vi "exec.vi"(8 "error in (no error)":errorcluster, 9 "Save Data":bool, 10 "VISA":refnum<visa-resource-name>, 11 "ElectrometerController in":refnum<class "ElectrometerController.lvclass">) -> (0 "error out":errorcluster, 3 "ElectrometerController out":refnum<class "ElectrometerController.lvclass">)   [LabVIEW 2016, in "ElectrometerController.lvclass"]
uses:
  ElectrometerController.lvclass
  Test/Global 1.vi
  Electrometer/Electrometer.lvclass
  Electrometer/State/State.lvclass
panel:
  out "Error Message":string
  in  "ReadingRate (ms)":dbl
  out "Running":bool
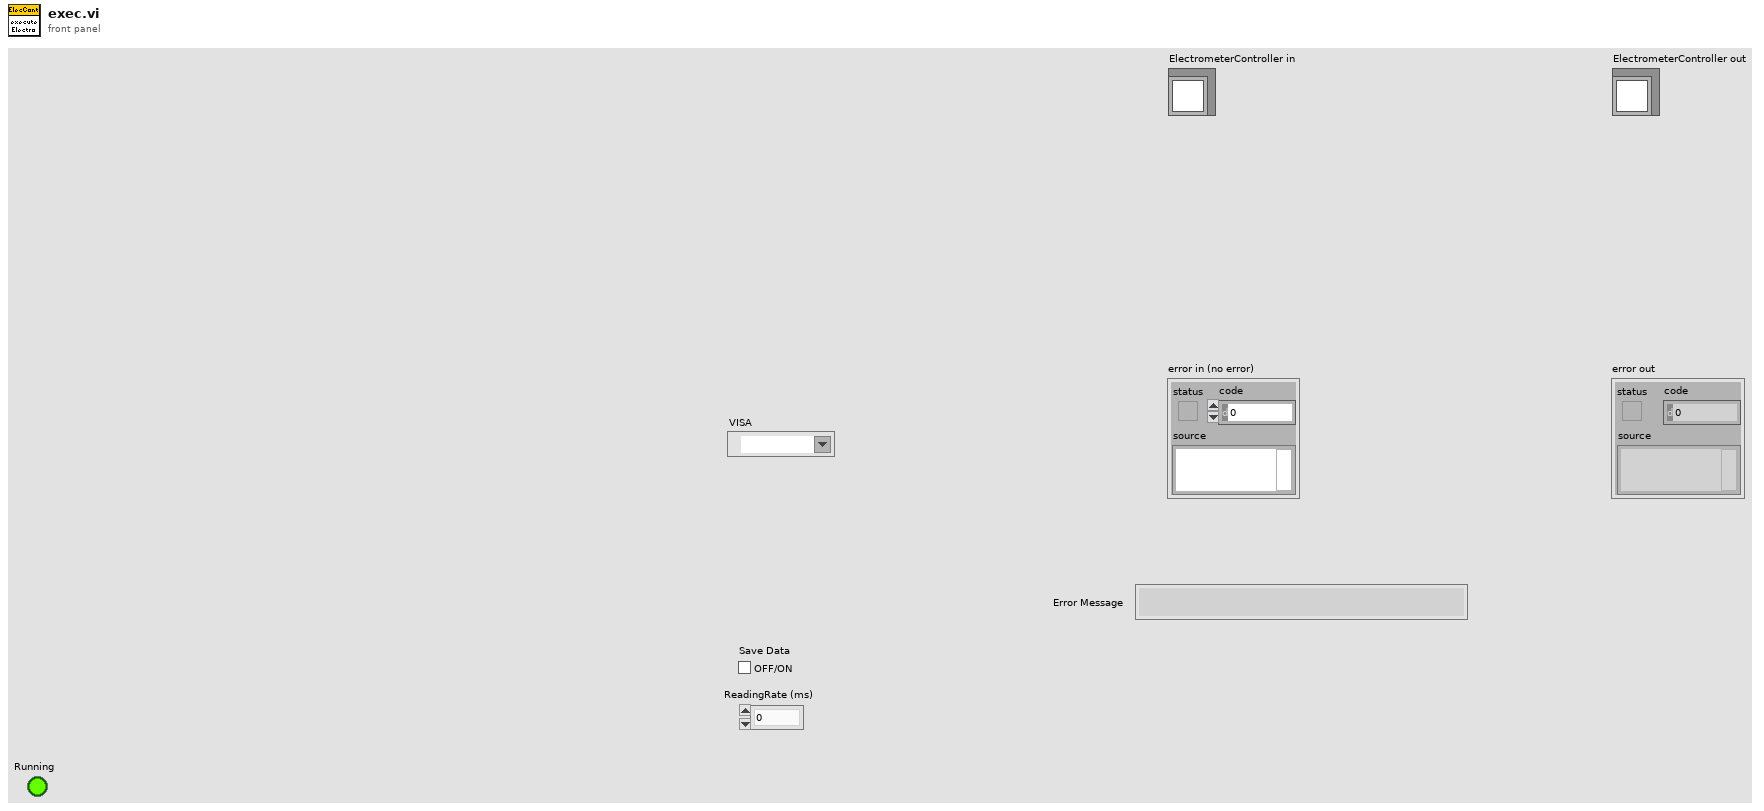
[diagram p1: front panel]
types:
  T1 = typedef "ElectrometerController.lvclass/functionalitiesEvnts.ctl" = cluster{"startManualRead":refnum<user-event>, "ChangeMeasure":refnum<user-event>, "startTimeRead":refnum<user-event>, "performZeroCalib":refnum<user-event>}
  T2 = cluster{"stopRead":refnum<user-event>, "stopApp":refnum<user-event>}
  T3 = typedef "Electrometer.lvclass/Modes.ctl" = i32
  T4 = typedef "ElectrometerError.lvclass/errorType.ctl" = cluster{"errorType":enum16{"Error", "Warning", "None"}, "errorCode":dbl, "hwError":string, "salError":string}
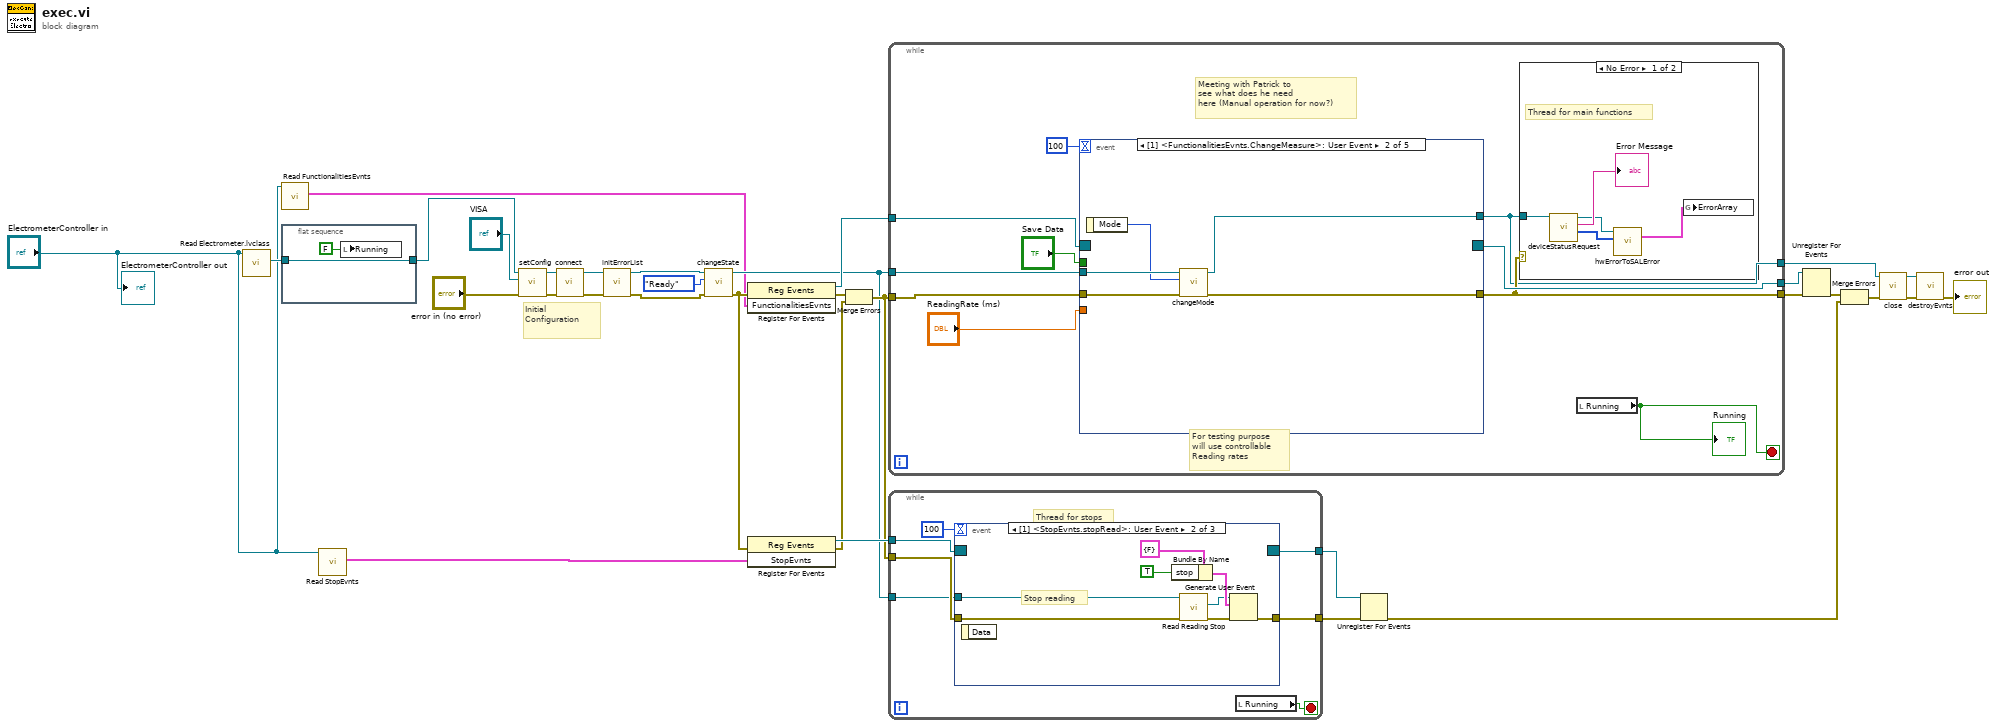
[diagram p0: block diagram]
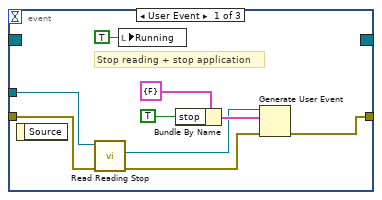
[diagram p2: hidden frame]
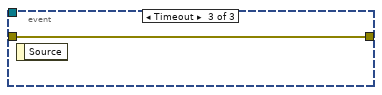
[diagram p3: hidden frame]
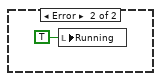
[diagram p4: hidden frame]
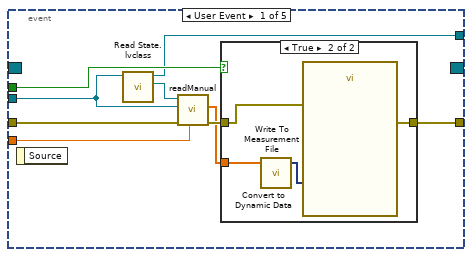
[diagram p5: hidden frame]
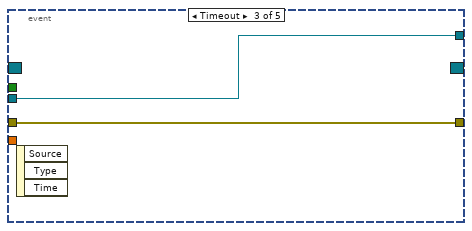
[diagram p7: hidden frame]
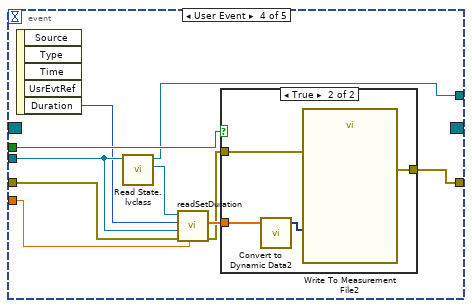
[diagram p8: hidden frame]
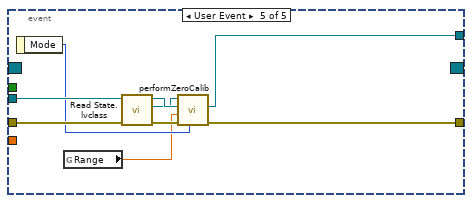
[diagram p10: hidden frame]
diagram:
  # "Initial Configuration"
  n1 = call-dynamic "Read Electrometer.lvclass.vi"("ElectrometerController in"="ElectrometerController in") -> ("Electrometer.lvclass"=w10:refnum<class "Electrometer.lvclass">)  [unwired: 8 in, 2 out]
  n2 = call-dynamic "Read FunctionalitiesEvnts.vi"("ElectrometerController in"="ElectrometerController in") -> ("FunctionalitiesEvnts"=w5:T1)  [unwired: 8 in, 2 out]
  n3 = flat-sequence {
    tunnel: w10 -> [w34]
    tunnel: [w34] -> w31
    frame #0 {
      n4 = local write "Running"(FALSE ("Running")) -> ()
    }
  }
  n5 = call-dynamic "Read StopEvnts.vi"("ElectrometerController in"="ElectrometerController in") -> ("StopEvnts"=w9:T2)  [unwired: 8 in, 2 out]
  n6 = call-dynamic "setConfig.vi"("error in (no error)"="error in (no error)", "VISA"="VISA", "Electrometer in"=w31) -> ("error out"=w29:errorcluster, "Electrometer out"=w28:refnum<class "Electrometer.lvclass">)  [unwired: 7 in]
  n7 = call "connect.vi"("error in (no error)"=w29, "Electrometer in"=w28) -> ("error out"=w4:errorcluster, "Electrometer out"=w3:refnum<class "Electrometer.lvclass">)  [unwired: 7 in, 1 out]
  n8 = call-dynamic "initErrorList.vi"("error in (no error)"=w4, "Electrometer in"=w3) -> ("error out"=w1:errorcluster, "Electrometer out"=w2:refnum<class "Electrometer.lvclass">)  [unwired: 8 in]
  n9 = call-dynamic "changeState.vi"("error in (no error)"=w1, "State"=enum16{"Configuring", "Ready", "Reading"}."Ready" ("newState"), "Electrometer in"=w2) -> ("error out"=w7:errorcluster, "Electrometer out"=w8:refnum<class "Electrometer.lvclass">)  [unwired: 7 in]
  n10 = register-events(error in=w7, w5) -> (reference out=w15:refnum<event-registration>, error out=w17:errorcluster)  [unwired: 1 in]
  n11 = register-events(error in=w7, w9) -> (reference out=w18:refnum<event-registration>, error out=w16:errorcluster)  [unwired: 1 in]
  n12 = Merge Errors(w17, w16) -> (w14:errorcluster)
  n13 = while {
    tunnel: w8 -> [w42]
    tunnel: w14 -> [w44]
    tunnel: [w38] -> w23
    tunnel: [w43] -> w24
    tunnel: [w35] -> w19
    tunnel: w15 -> [w39]
    stop <- w37 stop-if-true
    # "Thread for main functions"
    # "Meeting with Patrick to \nsee what does he need \nhere (Manual operation for now?)"
    # "For testing purpose\nwill use controllable \nReading rates"
    n14 = event shown="[1] <FunctionalitiesEvnts.ChangeMeasure>: User Event" {
      selector: w39 -> [_ _ _ _ _]
      dyn-events: [_ _ _ _ _] -> w43
      timeout: 100 -> [_ _ _ _ _]
      tunnel: w42 -> [w58 w66 w71 w79 w95]
      tunnel: w44 -> [w59 w69 w70 w81 w94]
      tunnel: [w55 w68 w70 w77 w89] -> w38
      tunnel: "Save Data" -> [w54 _ _ w78 _]
      tunnel: [w52 w67 w71 w74 w88] -> w35
      tunnel: "ReadingRate (ms)" -> [w51 _ _ w72 _]
      event User Event {
        n15 = event-data() -> ()  [unwired: 1 in, 1 out]
        n16 = call-dynamic "Read State.lvclass.vi"("Electrometer in"=w58) -> ("State.lvclass"=w57:refnum<class "State.lvclass">, "Electrometer out"=w52:refnum<class "Electrometer.lvclass">)  [unwired: 8 in, 1 out]
        n17 = call-dynamic "readManual.vi"("milliseconds to wait"=w51, "error in (no error)"=w59, "Electrometer in"=w58, "State in"=w57) -> ("error out"=w56:errorcluster, "results"=w53:dbl[])  [unwired: 4 in, 2 out]
        n18 = case shown="True" w54 {
          tunnel: [w60 w62] -> w55
          tunnel: w53 -> [_ w64]
          tunnel: w56 -> [w60 w61]
          frame False {
          }
          frame True {
            n19 = call "Convert to Dynamic Data"("Array"=w64) -> ("Dynamic Data Type"=w63:dynamicdata)  [unwired: 3 in]
            n20 = call "Write To Measurement File"("Signals"=w63, "error in (no error)"=w61) -> ("error out"=w62:errorcluster)  [unwired: 15 in, 2 out]
          }
        }
      }
      event User Event {
        n21 = event-data() -> ("Mode"=w65:T3)  [unwired: 1 in]
        n22 = call "changeMode.vi"("error in (no error)"=w69, "Measurement"=w65, "Electrometer in"=w66) -> ("error out"=w68:errorcluster, "Electrometer out"=w67:refnum<class "Electrometer.lvclass">)  [unwired: 7 in]
      }
      event Timeout {
        n23 = event-data() -> ()  [unwired: 1 in, 3 out]
      }
      event User Event {
        n24 = event-data() -> ("Duration"=w73:i32)  [unwired: 1 in, 4 out]
        n25 = call-dynamic "Read State.lvclass.vi"("Electrometer in"=w79) -> ("State.lvclass"=w80:refnum<class "State.lvclass">, "Electrometer out"=w74:refnum<class "Electrometer.lvclass">)  [unwired: 8 in, 1 out]
        n26 = call-dynamic "readSetDuration.vi"("loop delay"=w72, "error in (no error)"=w81, "Electrometer in"=w79, "duration"=w73, "State in"=w80) -> ("error out"=w75:errorcluster, "results"=w76:dbl[])  [unwired: 3 in, 2 out]
        n27 = case shown="True" w78 {
          tunnel: [w82 w84] -> w77
          tunnel: w76 -> [_ w86]
          tunnel: w75 -> [w82 w83]
          frame False {
          }
          frame True {
            n28 = call "Convert to Dynamic Data2"("Array"=w86) -> ("Dynamic Data Type"=w85:dynamicdata)  [unwired: 3 in]
            n29 = call "Write To Measurement File2"("Signals"=w85, "error in (no error)"=w83) -> ("error out"=w84:errorcluster)  [unwired: 15 in, 2 out]
          }
        }
      }
      event User Event {
        n30 = event-data() -> ("Mode"=w92:T3)  [unwired: 1 in]
        n31 = global read "Global 1.vi" "Range"() -> (w87:dbl)
        n32 = call-dynamic "Read State.lvclass.vi"("error in (no error)"=w94, "Electrometer in"=w95) -> ("error out"=w93:errorcluster, "State.lvclass"=w90:refnum<class "State.lvclass">, "Electrometer out"=w91:refnum<class "Electrometer.lvclass">)  [unwired: 7 in]
        n33 = call-dynamic "performZeroCalib.vi"("Mode"=w92, "error in (no error)"=w93, "Input Range"=w87, "Electrometer in"=w91, "State in"=w90) -> ("error out"=w89:errorcluster, "Electrometer out"=w88:refnum<class "Electrometer.lvclass">)  [unwired: 3 in, 2 out]
      }
    }
    n34 = case shown="No Error" w38 {
      tunnel: w35 -> [w49 _]
      frame No Error {
        n35 = call "deviceStatusRequest.vi"("Electrometer in"=w49) -> ("Device Code"=w46:i32[], "Error Message"=→"Error Message":string, "Electrometer out"=w47:refnum<class "Electrometer.lvclass">)  [unwired: 7 in, 1 out]
        n36 = call-dynamic "hwErrorToSALError.vi"("Error Code"=w46, "Electrometer in"=w47) -> ("ErrorArray"=w45:T4[])  [unwired: 7 in, 2 out]
        n37 = global write "Global 1.vi" "ErrorArray"(w45) -> ()
      }
      frame Error {
        n38 = local write "Running"(TRUE ("Running")) -> ()
      }
    }
    n39 = local read "Running"() -> (w37:bool)
    "Running" <- w37
  }
  n40 = while {
    tunnel: w18 -> [w102]
    tunnel: w14 -> [w99]
    tunnel: [w101] -> w27
    tunnel: [w100] -> w26
    tunnel: w8 -> [w98]
    stop <- w96 stop-if-true
    # "Thread for stops"
    n41 = event shown="[1] <StopEvnts.stopRead>: User Event" {
      selector: w102 -> [_ _ _]
      dyn-events: [_ _ _] -> w101
      timeout: 100 -> [_ _ _]
      tunnel: [w106 w114 w120] -> w100
      tunnel: w99 -> [w104 w112 w120]
      tunnel: w98 -> [w105 w113 _]
      event User Event {
        # "Stop reading + stop application"
        n42 = event-data() -> ()  [unwired: 1 in, 1 out]
        n43 = call-dynamic "Read Reading Stop.vi"("error in (no error)"=w104, "Electrometer in"=w105) -> ("error out"=w111:errorcluster, "ReadingStop"=w107:refnum<user-event>)  [unwired: 7 in, 1 out]
        n44 = local write "Running"(TRUE ("Running")) -> ()
        n45 = Bundle By Name(cluster=cluster{"stop":bool} {"stop"=FALSE} ("event data"), "stop"=TRUE) -> (w108:cluster{"stop":bool})
        n46 = Generate User Event(user event=w107, event data cluster=w108, error in=w111) -> (error out=w106:errorcluster)  [unwired: 1 in, 1 out]
      }
      event User Event {
        # "Stop reading"
        n47 = event-data() -> ()  [unwired: 1 in, 1 out]
        n48 = Bundle By Name(cluster=cluster{"stop":bool} {"stop"=FALSE} ("event data"), "stop"=TRUE) -> (w116:cluster{"stop":bool})
        n49 = call-dynamic "Read Reading Stop.vi"("error in (no error)"=w112, "Electrometer in"=w113) -> ("error out"=w119:errorcluster, "ReadingStop"=w115:refnum<user-event>)  [unwired: 7 in, 1 out]
        n50 = Generate User Event(user event=w115, event data cluster=w116, error in=w119) -> (error out=w114:errorcluster)  [unwired: 1 in, 1 out]
      }
      event Timeout {
        n51 = event-data() -> ()  [unwired: 1 in, 1 out]
      }
    }
    n52 = local read "Running"() -> (w96:bool)
  }
  n53 = Unregister For Events(event registration refnum=w27, error in=w26) -> (error out=w13:errorcluster)
  n54 = Unregister For Events(event registration refnum=w24, error in=w23) -> (error out=w25:errorcluster)
  n55 = Merge Errors(w25, w13) -> (w22:errorcluster)
  n56 = call "close.vi"("error in (no error)"=w22, "Electrometer in"=w19) -> ("error out"=w21:errorcluster, "Electrometer out"=w20:refnum<class "Electrometer.lvclass">)  [unwired: 8 in]
  n57 = call-dynamic "destroyEvnts.vi"("error in (no error)"=w21, "Electrometer in"=w20) -> ("error out"=→"error out":errorcluster)  [unwired: 8 in, 1 out]
  "ElectrometerController out" <- "ElectrometerController in"
